vi "ID_Connection_2.0.vi"() -> (2 "Arduino Uno":refnum<visa-resource-name>, 3 "Arduino Uno":string, 4 "Arduino Uno":bool, 6 "Pump":refnum<visa-resource-name>, 8 "Pump":string, 10 "Pump":bool, 13 "Arduino Mega":bool, 14 "Arduino Mega":string, 15 "Arduino Mega":refnum<visa-resource-name>)   [LabVIEW 2024]
uses:
  <vilib>/Instr/_visa.llb/VISA Find Search Mode.ctl
  154e74cf-856d-46b8-b8e9-1ea27d1d26b1.vi
  62d40bb6-eb46-4c2a-b9a7-6b4029ac7ca3.vi
  <vilib>/regexp/Match Regular Expression.xnode
panel:
  out "Array 2":bool[](array[boolean])
  out "Numeric":i32
  out "Array":string[](array[string])
  in  "error in":errorcluster
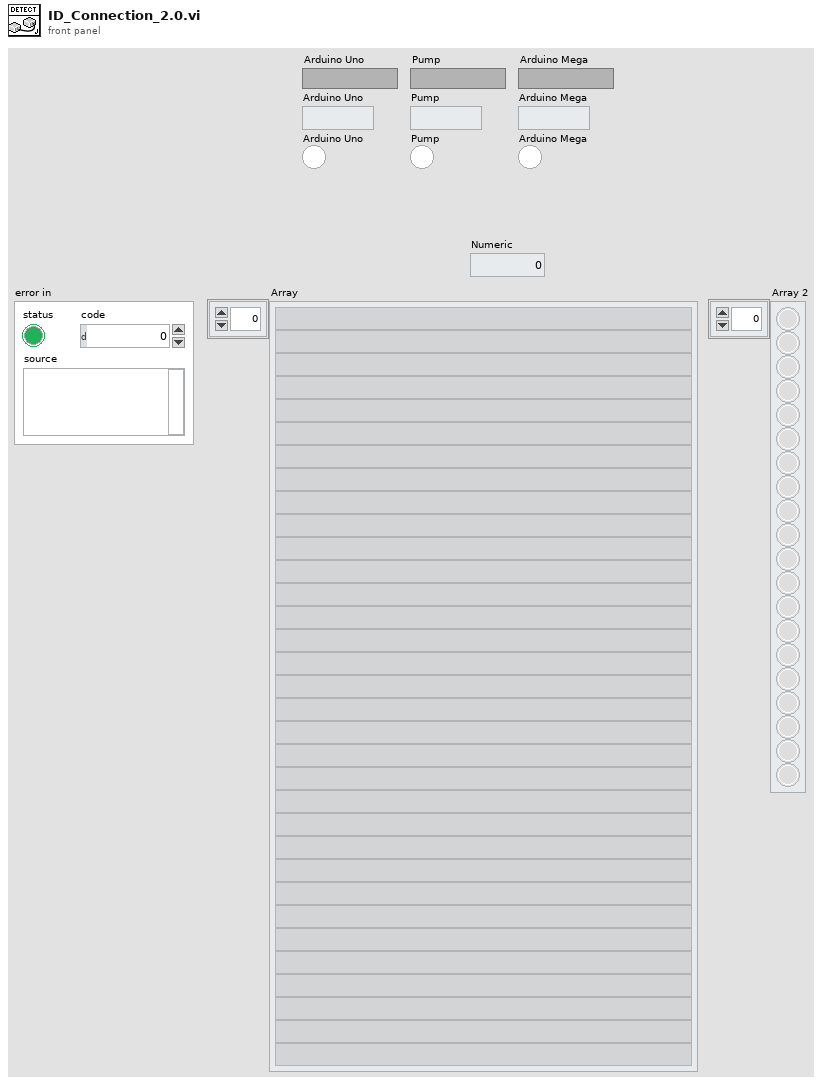
[diagram p1: front panel]
types:
  T1 = cluster{"VISA resource name":refnum<visa-resource-name>, "error out":errorcluster, "String":string}
  T2 = typedef "VISA Find Search Mode.ctl" = u32
  T3 = cluster{"VISA resource name":refnum<visa-resource-name>, "error out":errorcluster, string}
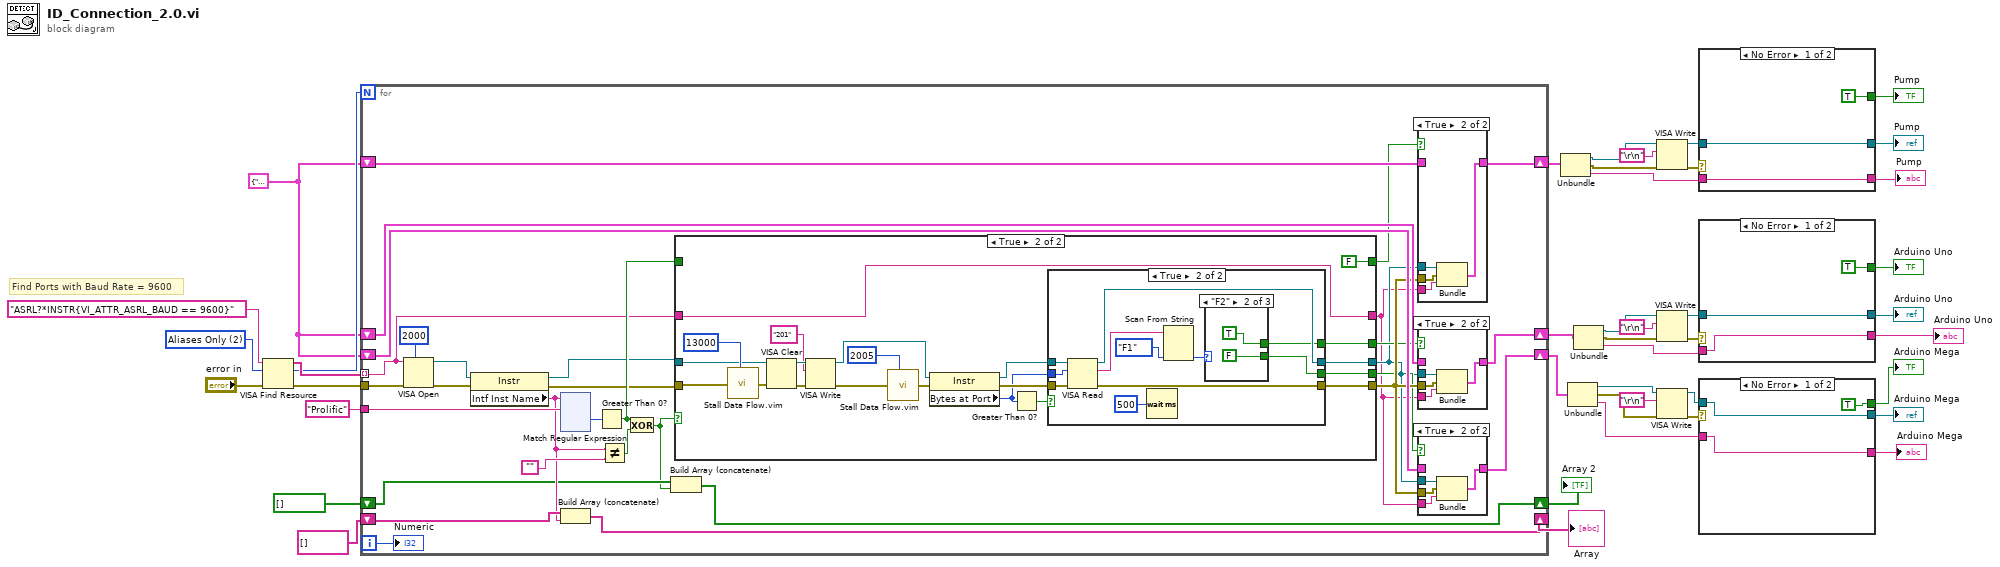
[diagram p0: block diagram]
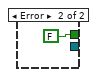
[diagram p2: hidden frame]
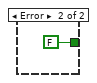
[diagram p3: hidden frame]
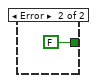
[diagram p4: hidden frame]
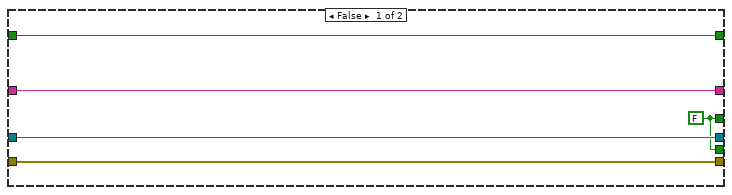
[diagram p6: hidden frame]
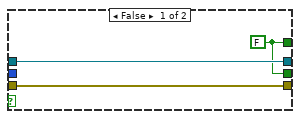
[diagram p7: hidden frame]
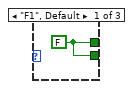
[diagram p8: hidden frame]
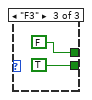
[diagram p9: hidden frame]
diagram:
  w16 = T1 {"VISA resource name"="", "error out"={"status"=FALSE, "code"=0, "source"=""}, "String"=""} ("Cluster")
  w39 = T2 2 items=["Canonical Names Only"=0, "Aliases Only"=2, "Include Matching Aliases"=3, "Include All Aliases"=4] ("Search Mode")
  # "Find Ports with Baud Rate = 9600"
  n1 = VISA Find Resource(8:"error in", 10:w39, 11:"ASRL?*INSTR{VI_ATTR_ASRL_BAUD == 9600}" ("expression (\"?*\")")) -> (0:w41:errorcluster, 2:w26:u32, 3:w42:string[])
  n2 = for {
    N: w26 -> [_]
    tunnel: w42 -> [w45] mode=indexing
    shift-right: [w72] -> w7
    shift-left: w16 -> [w71]
    tunnel: w41 -> [w70]
    shift-right: [w43] -> w15
    shift-left: w16 -> [w69]
    tunnel: "Prolific" -> [w67]
    shift-right: [w65] -> w25
    shift-left: string[] [] -> [w50]
    shift-right: [w64] -> w11
    shift-left: w16 -> [w63]
    shift-right: [w56] -> w19
    shift-left: bool[] [] -> [w48]
    i -> [w57]
    n3 = VISA Open(timeout (0)=u32 2000 ("VISA Open timeout (0)"), error in (no error)=w70, VISA resource name=w45) -> (VISA resource name=w73:refnum<visa-resource-name>, error out=w52:errorcluster)  [unwired: 2 in]
    n4 = property class="Instr"(reference=w73, error in=w52) -> (reference out=w51:refnum<visa-resource-name>, error out=w46:errorcluster, "Intf Inst Name"=w49:string)
    n5 = xnode "Match Regular Expression"("input string"=w49, "regular expression"=w67) -> ("offset past match"=w68:i32)  [unwired: 4 in, 4 out]
    n6 = Build Array (concatenate)(w50, w49) -> (w65:string[])
    n7 = Greater Than 0?(x=w68) -> (x > 0?=w53:bool)
    n8 = Not Equal?(x=w49, y="") -> (x != y?=w54:bool)
    n9 = Exclusive Or(1:w54, 2:w53) -> (0:w47:bool)
    n10 = Build Array (concatenate)(w48, w47) -> (w56:bool[])
    n11 = case shown="True" w47 {
      tunnel: w51 -> [w83 w86]
      tunnel: w46 -> [w82 w85]
      tunnel: [w83 w97] -> w59
      tunnel: [w82 w96] -> w62
      tunnel: [w81 w94] -> w61
      tunnel: [w81 w95] -> w60
      tunnel: [w80 FALSE] -> w58
      tunnel: w53 -> [w80 _]
      tunnel: w45 -> [w79 w84]
      tunnel: [w79 w84] -> w44
      frame False {
        w81 = FALSE
      }
      frame True {
        n12 = call "Stall Data Flow.vim"("value in"=w85, "milliseconds to wait"=u32 13000) -> ("value out"=w88:errorcluster)  [unwired: 1 out]
        n13 = VISA Clear(VISA resource name=w86, error in (no error)=w88) -> (VISA resource name out=w103:refnum<visa-resource-name>, error out=w104:errorcluster)
        n14 = VISA Write(VISA resource name=w103, write buffer="201", error in (no error)=w104) -> (VISA resource name out=w101:refnum<visa-resource-name>, error out=w92:errorcluster)  [unwired: 1 out]
        n15 = call "Stall Data Flow.vim"("value in"=w92, "milliseconds to wait"=u32 2005) -> ("value out"=w91:errorcluster)  [unwired: 1 out]
        n16 = property class="Instr"(reference=w101, error in=w91) -> (reference out=w99:refnum<visa-resource-name>, error out=w98:errorcluster, "Bytes at Port"=w93:u32)
        n17 = Greater Than 0?(x=w93) -> (x > 0?=w100:bool)
        n18 = case shown="True" w100 {
          tunnel: w99 -> [w107 w118]
          tunnel: w98 -> [w106 w117]
          tunnel: [w107 w116] -> w97
          tunnel: [w106 w115] -> w96
          tunnel: [w105 w113] -> w95
          tunnel: [w105 w114] -> w94
          tunnel: w93 -> [_ w109]
          frame False {
            w105 = FALSE
          }
          frame True {
            n19 = VISA Read(VISA resource name=w118, byte count=w109, error in (no error)=w117) -> (VISA resource name out=w116:refnum<visa-resource-name>, read buffer=w112:string, error out=w115:errorcluster)  [unwired: 1 out]
            n20 = Wait (ms)(milliseconds to wait=u32 500) -> ()  [unwired: 1 out]
            n21 = Scan From String(input string=w112, default 1=enum16{"F1", "F2", "F3"}."F1") -> (output 1=w110:enum16{"F1", "F2", "F3"})  [unwired: 3 in, 3 out]
            n22 = case shown="\"F2\"" w110 {
              tunnel: [w119 FALSE TRUE] -> w114
              tunnel: [w119 TRUE FALSE] -> w113
              frame "F1", Default {
                w119 = FALSE
              }
              frame "F2" {
              }
              frame "F3" {
              }
            }
          }
        }
      }
    }
    n23 = case shown="True" w58 {
      tunnel: w59 -> [_ w245]
      tunnel: w62 -> [_ w244]
      tunnel: [w241 w243] -> w43
      tunnel: w69 -> [w241 _]
      tunnel: w44 -> [_ w242]
      frame False {
      }
      frame True {
        n24 = Bundle("VISA resource name"=w245, "error out"=w244, w242) -> (w243:T3)  [unwired: 1 in]
      }
    }
    n25 = case shown="True" w60 {
      tunnel: w59 -> [_ w250]
      tunnel: w62 -> [_ w249]
      tunnel: [w246 w248] -> w72
      tunnel: w71 -> [w246 _]
      tunnel: w44 -> [_ w247]
      frame False {
      }
      frame True {
        n26 = Bundle("VISA resource name"=w250, "error out"=w249, w247) -> (w248:T3)  [unwired: 1 in]
      }
    }
    n27 = case shown="True" w61 {
      tunnel: w59 -> [_ w78]
      tunnel: w62 -> [_ w77]
      tunnel: [w74 w76] -> w64
      tunnel: w63 -> [w74 _]
      tunnel: w44 -> [_ w75]
      frame False {
      }
      frame True {
        n28 = Bundle("VISA resource name"=w78, "error out"=w77, w75) -> (w76:T3)  [unwired: 1 in]
      }
    }
    "Numeric" <- w57
  }
  "Array" <- w25
  "Array 2" <- w19
  n29 = Unbundle(w15) -> ("VISA resource name"=w14:refnum<visa-resource-name>, "error out"=w13:errorcluster, "String"=w12:string)
  n30 = Unbundle(w11) -> ("VISA resource name"=w10:refnum<visa-resource-name>, "error out"=w9:errorcluster, "String"=w8:string)
  n31 = Unbundle(w7) -> ("VISA resource name"=w6:refnum<visa-resource-name>, "error out"=w5:errorcluster, "String"=w4:string)
  n32 = VISA Write(VISA resource name=w14, write buffer="\r\n", error in (no error)=w13) -> (VISA resource name out=w31:refnum<visa-resource-name>, error out=w33:errorcluster)  [unwired: 1 out]
  n33 = VISA Write(VISA resource name=w6, write buffer="\r\n", error in (no error)=w5) -> (VISA resource name out=w37:refnum<visa-resource-name>, error out=w36:errorcluster)  [unwired: 1 out]
  n34 = VISA Write(VISA resource name=w10, write buffer="\r\n", error in (no error)=w9) -> (VISA resource name out=w20:refnum<visa-resource-name>, error out=w21:errorcluster)  [unwired: 1 out]
  n35 = case shown="No Error" w33 {
    tunnel: [w253 _] -> w32
    tunnel: w31 -> [w253 _]
    tunnel: [TRUE FALSE] -> w30
    tunnel: w12 -> [w251 _]
    tunnel: [w251 _] -> w3
    frame No Error {
    }
    frame Error {
    }
  }
  "Pump" <- w32
  "Pump" <- w30
  "Pump" <- w3
  n36 = case shown="No Error" w36 {
    tunnel: [TRUE FALSE] -> w34
    tunnel: w37 -> [w256 _]
    tunnel: [w256 _] -> w35
    tunnel: w4 -> [w255 _]
    tunnel: [w255 _] -> w2
    frame No Error {
    }
    frame Error {
    }
  }
  "Arduino Uno" <- w35
  "Arduino Uno" <- w34
  "Arduino Uno" <- w2
  n37 = case shown="No Error" w21 {
    tunnel: [TRUE FALSE] -> w23
    tunnel: w20 -> [w260 _]
    tunnel: [w260 _] -> w22
    tunnel: w8 -> [w259 _]
    tunnel: [w259 _] -> w1
    frame No Error {
    }
    frame Error {
    }
  }
  "Arduino Mega" <- w22
  "Arduino Mega" <- w23
  "Arduino Mega" <- w1
